vi "Compare_Costs_101-11_F()_Rearrange_Indices-1.vi"(5 "[IN] Cost functions":i8[](array[numeric]), 7 "[IN] Subtracks":T1(array[cluster])) -> (2 "[OUT] Indicies of sub\ntracks for transforma\ntion (resolving)":i32[](array[numeric]))   [LabVIEW 2013]
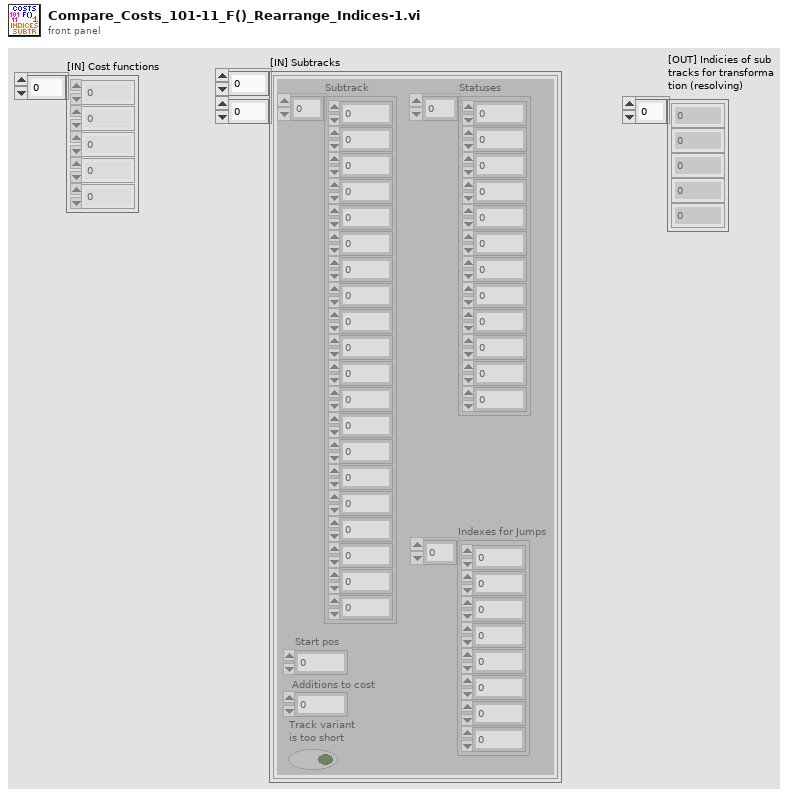
[diagram p1: front panel]
types:
  T1 = cluster{"Subtrack":dbl[], "Statuses":i16[], "Start pos":i32, "Additions to cost":i32, "Track variant \nis too short":bool, "Indexes for Jumps":i32[]}[][]
  T2 = cluster{"Subtrack":dbl[], "Statuses":i16[], "Start pos":i32, "Additions to cost":i32, "Track variant \nis too short":bool, "Indexes for Jumps":i32[]}[]
  T3 = cluster{"Subtrack":dbl[], "Statuses":i16[], "Start pos":i32, "Additions to cost":i32, "Track variant \nis too short":bool, "Indexes for Jumps":i32[]}
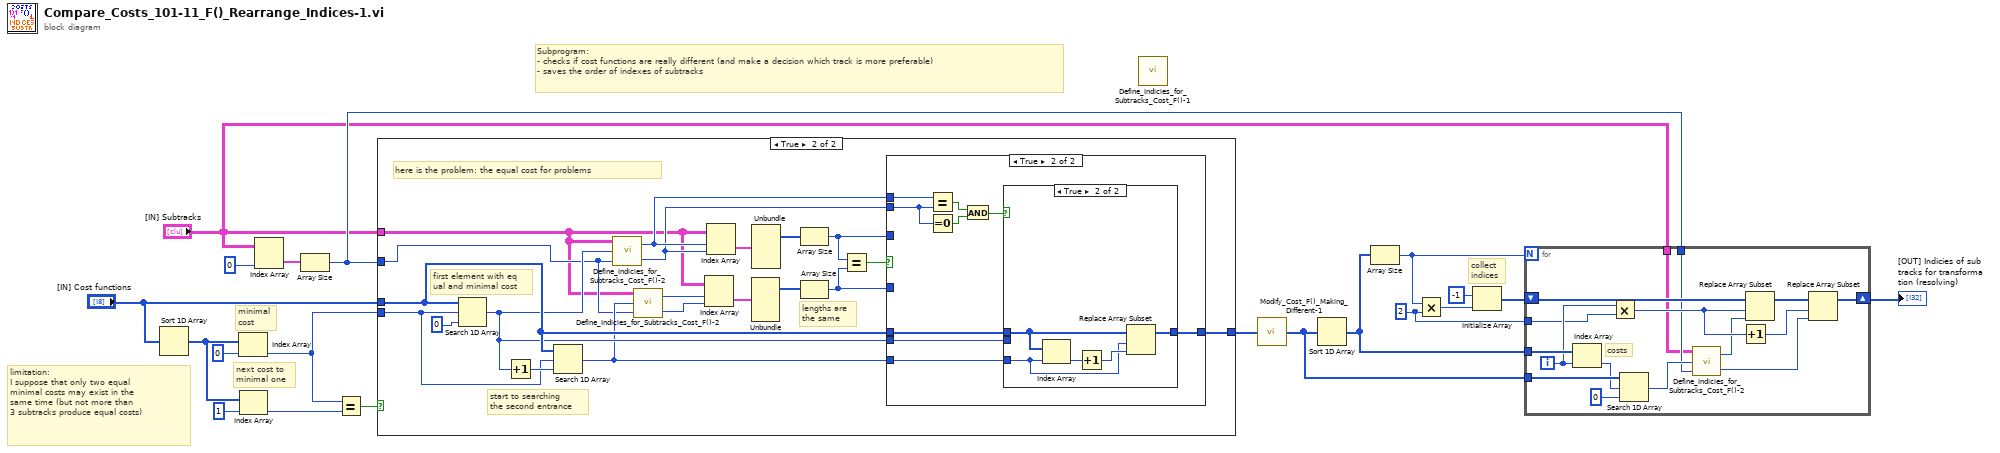
[diagram p0: block diagram]
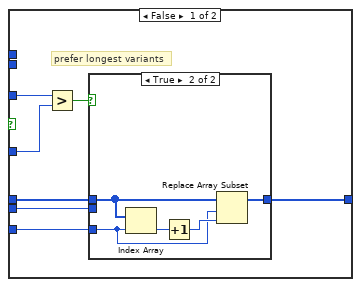
[diagram p3: hidden frame]
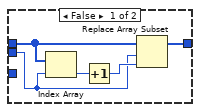
[diagram p4: hidden frame]
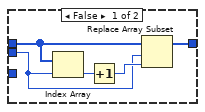
[diagram p5: hidden frame]
diagram:
  w5 = 2 ("y")
  # "collect\nindices"
  # "limitation: \nI suppose that only two equal\nminimal costs may exist in the \nsame time (but not more than\n3 subtracks produce equal costs)"
  # "next cost to \nminimal one"
  # "minimal\ncost"
  # "Subprogram:\n- checks if cost functions are really different (and make a decision which track is more preferable)\n- saves the order of indexes of subtracks"
  n1 = Sort 1D Array(array="[IN] Cost functions") -> (sorted array=w16:i8[])
  n2 = Index Array(array=w16, index=0) -> (element=w15:i8)
  n3 = Index Array(array=w16, index=1) -> (element=w18:i8)
  n4 = Index Array(array="[IN] Subtracks", index (col)=0 ("disabled index (col)")) -> (element=w8:T2)  [unwired: 1 in]
  n5 = Array Size(array=w8) -> (size(s)=w4:i32)
  n6 = Equal?(x=w15, y=w18) -> (x = y?=w17:bool)
  n7 = case shown="True" w17 {
    tunnel: "[IN] Subtracks" -> [_ w22]
    tunnel: "[IN] Cost functions" -> [w21 w33]
    tunnel: w15 -> [_ w39]
    tunnel: [w21 w30] -> w2
    tunnel: w4 -> [_ w25]
    frame False {
    }
    frame True {
      # "lengths are\nthe same"
      # "start to searching\nthe second entrance"
      # "first element with eq\nual and minimal cost"
      # "here is the problem: the equal cost for problems"
      n8 = Search 1D Array(1D array=w33, element=w39, start index (0)=0) -> (index of element=w29:i32)
      n9 = Increment(x=w29) -> (x+1=w40:i32)
      n10 = Search 1D Array(1D array=w33, element=w39, start index (0)=w40) -> (index of element=w26:i32)
      n11 = call "Define_Indicies_for_Subtracks_Cost_F()-2.vi"("[IN] Number of Rows"=w25, "[IN] Current index"=w29, "[IN] Subtracks"=w22) -> ("[OUT] Column \n# for Subtrack"=w27:i32, "[OUT] Row # \nfor Subtrack"=w28:i32)
      n12 = call "Define_Indicies_for_Subtracks_Cost_F()-2.vi"("[IN] Number of Rows"=w25, "[IN] Current index"=w26, "[IN] Subtracks"=w22) -> ("[OUT] Column \n# for Subtrack"=w23:i32, "[OUT] Row # \nfor Subtrack"=w24:i32)
      n13 = Index Array(array=w22, index (row)=w24, index (col)=w23) -> (element=w37:T3)
      n14 = Index Array(array=w22, index (row)=w28, index (col)=w27) -> (element=w38:T3)
      n15 = Unbundle(w37) -> ("Statuses"=w35:i16[])  [unwired: 5 out]
      n16 = Unbundle(w38) -> ("Statuses"=w36:i16[])  [unwired: 5 out]
      n17 = Array Size(array=w36) -> (size(s)=w32:i32)
      n18 = Array Size(array=w35) -> (size(s)=w31:i32)
      n19 = Equal?(x=w32, y=w31) -> (x = y?=w34:bool)
      n20 = case shown="True" w34 {
        tunnel: w33 -> [w45 w67]
        tunnel: [w42 w66] -> w30
        tunnel: w26 -> [w44 w65]
        tunnel: w29 -> [w43 w64]
        tunnel: w32 -> [w48 _]
        tunnel: w31 -> [w47 _]
        tunnel: w28 -> [_ w63]
        tunnel: w27 -> [_ w62]
        frame False {
          # "prefer longest variants"
          n21 = Greater?(x=w48, y=w47) -> (0:w46:bool)
          n22 = case shown="True" w46 {
            tunnel: w45 -> [w51 w57]
            tunnel: [w50 w55] -> w42
            tunnel: w44 -> [_ w54]
            tunnel: w43 -> [w49 _]
            frame False {
              n23 = Index Array(array=w51, index=w49) -> (element=w53:i8)
              n24 = Increment(x=w53) -> (x+1=w52:i8)
              n25 = Replace Array Subset(array=w51, new element=w52, index=w49) -> (w50:i8[])
            }
            frame True {
              n26 = Index Array(array=w57, index=w54) -> (element=w58:i8)
              n27 = Increment(x=w58) -> (x+1=w56:i8)
              n28 = Replace Array Subset(array=w57, new element=w56, index=w54) -> (w55:i8[])
            }
          }
        }
        frame True {
          n29 = Equal?(x=w63, y=w62) -> (x = y?=w60:bool)
          n30 = Equal To 0?(x=w62) -> (x = 0?=w61:bool)
          n31 = And(x=w60, y=w61) -> (x .and. y?=w59:bool)
          n32 = case shown="True" w59 {
            tunnel: w67 -> [w70 w76]
            tunnel: [w69 w74] -> w66
            tunnel: w65 -> [_ w73]
            tunnel: w64 -> [w68 _]
            frame False {
              n33 = Index Array(array=w70, index=w68) -> (element=w72:i8)
              n34 = Increment(x=w72) -> (x+1=w71:i8)
              n35 = Replace Array Subset(array=w70, new element=w71, index=w68) -> (w69:i8[])
            }
            frame True {
              n36 = Index Array(array=w76, index=w73) -> (element=w77:i8)
              n37 = Increment(x=w77) -> (x+1=w75:i8)
              n38 = Replace Array Subset(array=w76, new element=w75, index=w73) -> (w74:i8[])
            }
          }
        }
      }
    }
  }
  n39 = call "Define_Indicies_for_Subtracks_Cost_F()-1.vi"() -> ()  [unwired: 2 in, 2 out]
  n40 = call "Modify_Cost_F()_Making_Different-1.vi"("[IN] Cost functions"=w2) -> ("[OUT] Cost functions"=w1:i8[])
  n41 = Sort 1D Array(array=w1) -> (sorted array=w11:i8[])
  n42 = Array Size(array=w11) -> (size(s)=w7:i32)
  n43 = Multiply(x=w7, y=w5) -> (x*y=w6:i32)
  n44 = Initialize Array(-1 ("index"), w6) -> (w12:i32[])
  n45 = for {
    N: w7 -> [_]
    shift-right: [w84] -> w10
    shift-left: w12 -> [w89]
    tunnel: w11 -> [w93]
    tunnel: w1 -> [w92]
    tunnel: w5 -> [w87]
    tunnel: w4 -> [w79]
    tunnel: "[IN] Subtracks" -> [w78]
    i -> [w88]
    # "costs"
    n46 = Index Array(array=w93, index=w88) -> (element=w91:i8)
    n47 = Multiply(x=w88, y=w87) -> (x*y=w86:i32)
    n48 = Search 1D Array(1D array=w92, element=w91, start index (0)=0) -> (index of element=w80:i32)
    n49 = call "Define_Indicies_for_Subtracks_Cost_F()-2.vi"("[IN] Number of Rows"=w79, "[IN] Current index"=w80, "[IN] Subtracks"=w78) -> ("[OUT] Column \n# for Subtrack"=w81:i32, "[OUT] Row # \nfor Subtrack"=w82:i32)
    n50 = Increment(x=w86) -> (x+1=w83:i32)
    n51 = Replace Array Subset(array=w89, new element=w82, index=w86) -> (w85:i32[])
    n52 = Replace Array Subset(array=w85, new element=w81, index=w83) -> (w84:i32[])
  }
  "[OUT] Indicies of sub\ntracks for transforma\ntion (resolving)" <- w10
